vi "Configure Current Trigger.vi"(8 "error in (no error)":errorcluster, 9 "Current Trigger Slope (0: Positive)":u16(ring) items=["Positive", "Negative"], 10 "Current Trigger Level (0 A)":dbl, 11 "VISA resource name":refnum<visa-resource-name>) -> (0 "error out":errorcluster, 3 "VISA resource name out":refnum<visa-resource-name>)   [LabVIEW 2019, in "Agilent N7976A.lvlib"]
doc: "Configures the settings necessary for a current-based trigger."
uses:
  <instrlib>/Agilent N7976A/Agilent N7976A.lvlib
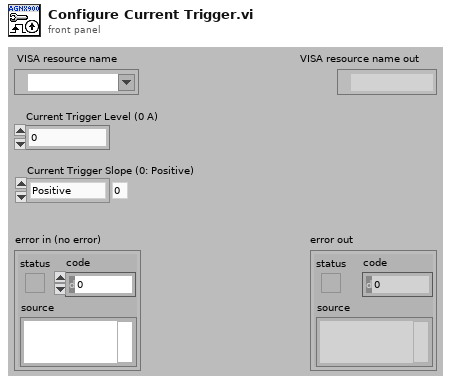
[diagram p1: front panel]
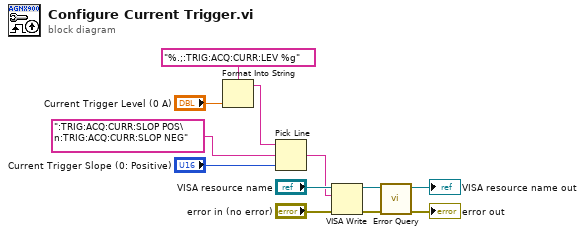
[diagram p0: block diagram]
diagram:
  n1 = Format Into String(format string="%.;:TRIG:ACQ:CURR:LEV %g", "Current Trigger Level (0 A)") -> (resulting string=w3:string)  [unwired: 2 in, 1 out]
  n2 = Pick Line(string ("")=w3, multi-line string=":TRIG:ACQ:CURR:SLOP POS\n:TRIG:ACQ:CURR:SLOP NEG" ("format string"), line index="Current Trigger Slope (0: Positive)") -> (output string=w4:string)
  n3 = VISA Write(VISA resource name="VISA resource name", write buffer=w4, error in (no error)="error in (no error)") -> (VISA resource name out=w10:refnum<visa-resource-name>, error out=w9:errorcluster)  [unwired: 1 out]
  n4 = call <instrlib>:"Error Query.vi"("error in (no error)"=w9, "VISA resource name"=w10) -> ("error out"=→"error out":errorcluster, "VISA resource name out"=→"VISA resource name out":refnum<visa-resource-name>)  [unwired: 6 in, 2 out]
